vi "Length.vi"(1 "Vec2 in":refnum<class "Vector2.lvclass">) -> (0 "Length out":dbl)   [LabVIEW 2022 SP3, in "Vector2.lvclass"]
uses:
  Vector2.lvclass
  Vector2.lvclass/Vector2.ctl
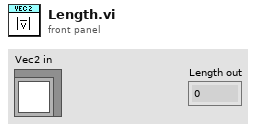
[diagram p1: front panel]
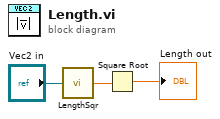
[diagram p0: block diagram]
diagram:
  n1 = call "LengthSqr.vi"("Vec2 in"="Vec2 in") -> ("Length Sqr out"=w2:dbl)
  n2 = Square Root(x=w2) -> (sqrt(x)=→"Length out":dbl)
